vi "create table.vi"(10 "error in":errorcluster) -> (2 "error out":errorcluster)   [LabVIEW 2017]
uses:
  Database/Controls/DB Options.ctl
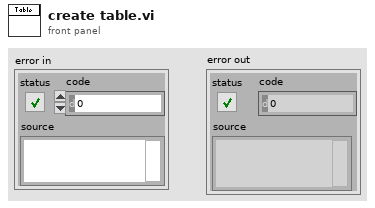
[diagram p1: front panel]
types:
  T1 = typedef "DB Options.ctl" = enum16{"Select", "Execute", "Special Q", "Insert", "Update", "Delete", "Open", "Close"}
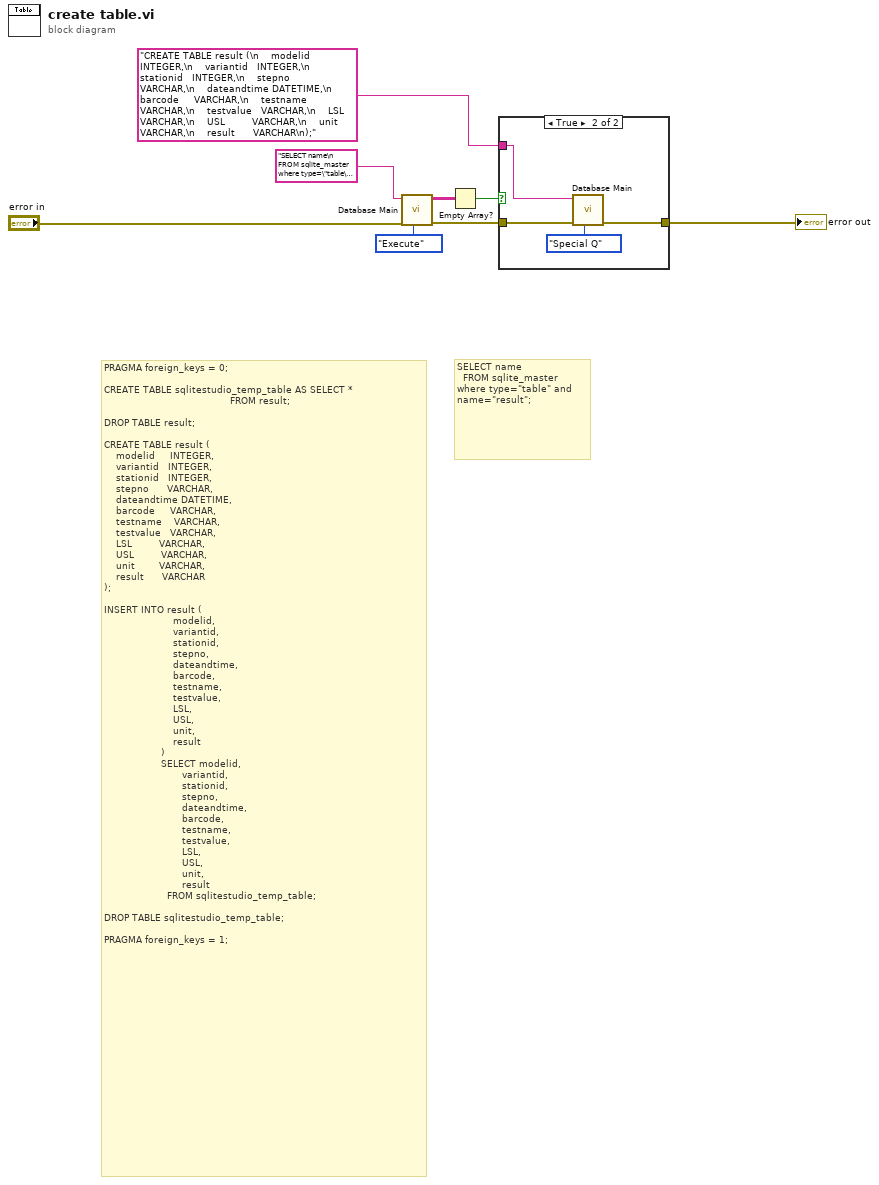
[diagram p0: block diagram]
diagram:
  # "SELECT name\n  FROM sqlite_master where type=\"table\" and name=\"result\";"
  # "PRAGMA foreign_keys = 0;\n\nCREATE TABLE sqlitestudio_temp_table AS SELECT *\n                                          FROM result;\n\nDROP TABLE result;\n\nCREATE TABLE result (\n    modelid     INTEGER,\n    variantid   INTEGER,\n    stationid   INTEGER,\n    stepno      VARCHAR,\n    dateandtime DATETIME,\n    barcode     VARCHAR,\n    testname    VARCHAR,\n    testvalue   VARCHAR,\n    LSL         VARCHAR,\n    USL         VARCHAR,\n    unit        VARCHAR,\n    result      VARCHAR\n);\n\nINSERT INTO result (\n                       modelid,\n                       variantid,\n                       stationid,\n                       stepno,\n                       dateandtime,\n                       barcode,\n                       testname,\n                       testvalue,\n                       LSL,\n                       USL,\n                       unit,\n                       result\n                   )\n                   SELECT modelid,\n                          variantid,\n                          stationid,\n                          stepno,\n                          dateandtime,\n                          barcode,\n                          testname,\n                          testvalue,\n                          LSL,\n                          USL,\n                          unit,\n                          result\n                     FROM sqlitestudio_temp_table;\n\nDROP TABLE sqlitestudio_temp_table;\n\nPRAGMA foreign_keys = 1;"
  n1 = call "Database Main.vi"("Option"=DB_Options."Execute", "error in (no error)"="error in", "table Name/Query"="SELECT name\n  FROM sqlite_master where type=\"table\" and name=\"result\";\n") -> ("error out"=w2:errorcluster, "Data"=w4:string[][])  [unwired: 6 in, 1 out]
  n2 = Empty Array?(array=w4) -> (empty?=w3:bool)
  n3 = case shown="True" w3 {
    tunnel: w2 -> [w9 w12]
    tunnel: [w9 w11] -> w8
    tunnel: "CREATE TABLE result (\n    modelid     INTEGER,\n    variantid   INTEGER,\n    stationid   INTEGER,\n    stepno      VARCHAR,\n    dateandtime DATETIME,\n    barcode     VARCHAR,\n    testname    VARCHAR,\n    testvalue   VARCHAR,\n    LSL         VARCHAR,\n    USL         VARCHAR,\n    unit        VARCHAR,\n    result      VARCHAR\n);" ("table Name/Query") -> [_ w10]
    frame False {
    }
    frame True {
      n4 = call "Database Main.vi"("Option"=DB_Options."Special Q", "error in (no error)"=w12, "table Name/Query"=w10) -> ("error out"=w11:errorcluster)  [unwired: 6 in, 2 out]
    }
  }
  "error out" <- w8
